vi "Read Next.vi"(8 "error in (no error)":errorcluster, 11 "ReadoutDevice in":refnum<class "ReadoutDevice.lvclass">) -> (0 "error out":errorcluster, 2 "Actor Framework:Message Enqueuer":refnum<class "Message Enqueuer.lvclass">, 3 "ReadoutDevice out":refnum<class "ReadoutDevice.lvclass">)   [LabVIEW 2013]
uses:
  ReadoutDevice.lvclass
  <vilib>/ActorFramework/Message Enqueuer/Message Enqueuer.lvclass
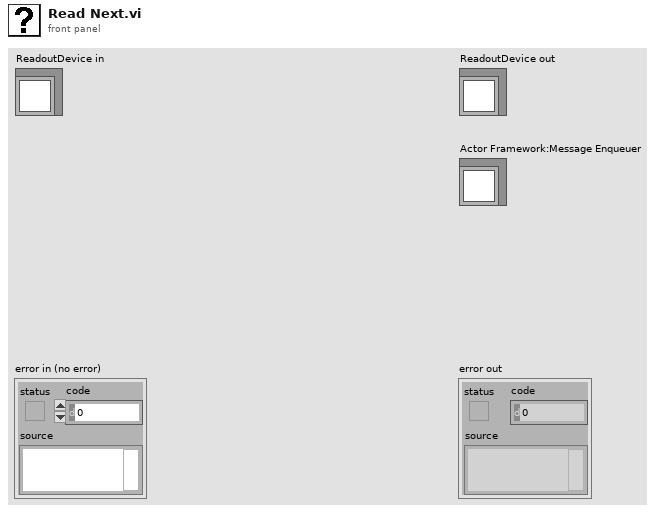
[diagram p1: front panel]
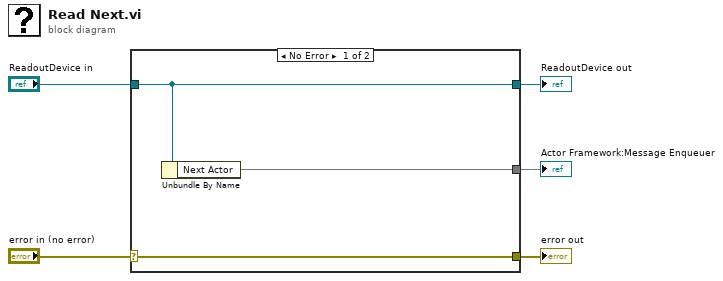
[diagram p0: block diagram]
diagram:
  n1 = case shown="No Error" "error in (no error)" {
    selector: "error in (no error)" -> [w8 w9]
    tunnel: [w8 w9] -> w4
    tunnel: [w7 w10] -> w2
    tunnel: "ReadoutDevice in" -> [w7 w10]
    tunnel: [w6 _] -> w1
    frame No Error {
      n2 = Unbundle By Name(w7) -> ("Next Actor"=w6)
    }
    frame Error {
    }
  }
  "error out" <- w4
  "ReadoutDevice out" <- w2
  "Actor Framework:Message Enqueuer" <- w1
